vi "NextMessage.vi"(6 "error in":errorcluster, 7 "timeout in ms (-1)":i32, 9 "message queue in":T1) -> (0 "error out":errorcluster, 1 "timed out?":bool, 2 "exit":bool, 3 "message queue out":T1, 4 "Value":string, 5 "Name":string)   [LabVIEW 2014, in "Raspberry Pi Compatible Compiler for LabVIEW.lvlib" / "SimpleMessaging.lvlib"]
uses:
  SimpleMessaging.lvlib
  MessageQueueTD.ctl
  MessageTD.ctl
  PackageMessage.vi
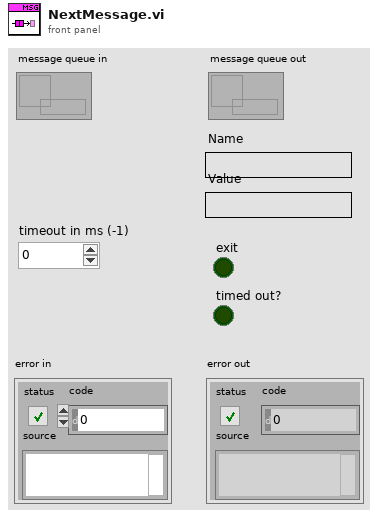
[diagram p1: front panel]
types:
  T1 = typedef "Raspberry Pi Compatible Compiler for LabVIEW.lvlib/SimpleMessaging.lvlib/MessageQueueTD.ctl" = refnum<queue>
  T2 = typedef "Raspberry Pi Compatible Compiler for LabVIEW.lvlib/SimpleMessaging.lvlib/MessageTD.ctl" = cluster{"Name":string, "Value":string}
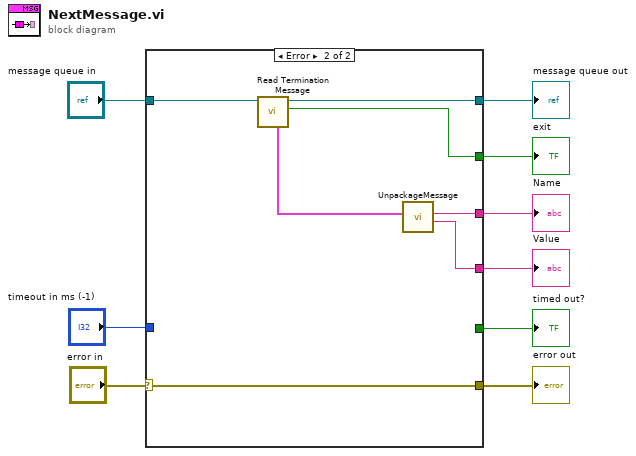
[diagram p0: block diagram]
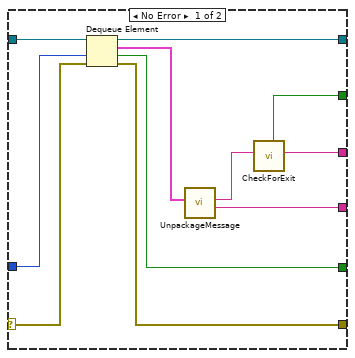
[diagram p2: hidden frame]
diagram:
  n1 = case shown="Error" "error in" {
    selector: "error in" -> [w10 w21]
    tunnel: "message queue in" -> [w20 w27]
    tunnel: "timeout in ms (-1)" -> [w19 _]
    tunnel: [w18 w26] -> w7
    tunnel: [w17 w21] -> w6
    tunnel: [w16 _] -> w5
    tunnel: [w14 w22] -> w4
    tunnel: [w12 w25] -> w3
    tunnel: [w11 w23] -> w2
    frame No Error {
      n2 = Dequeue Element(queue=w20, timeout in ms (-1)=w19, error in (no error)=w10) -> (queue out=w18:T1, element=w15:T2, timed out?=w16:bool, error out=w17:errorcluster)
      n3 = call "UnpackageMessage.vi"("Message"=w15) -> ("Value"=w14:string, "Name"=w13:string)  [unwired: 9 in]
      n4 = call "CheckForExit.vi"("Name"=w13) -> ("Name out"=w11:string, "exit"=w12:bool)  [unwired: 7 in]
    }
    frame Error {
      n5 = call "Read Termination Message.vi"("message queue in"=w27) -> ("termination message"=w25:bool, "message queue out"=w26:T1, "Message"=w24:T2)  [unwired: 6 in]
      n6 = call "UnpackageMessage.vi"("Message"=w24) -> ("Value"=w22:string, "Name"=w23:string)  [unwired: 9 in]
    }
  }
  "message queue out" <- w7
  "Name" <- w2
  "Value" <- w4
  "error out" <- w6
  "timed out?" <- w5
  "exit" <- w3
